vi "Switch - Making Connections on a Switch (NI-SWITCH).vi"() -> ()   [LabVIEW 2019]
doc: "I. Description:\n\nThis example demonstrates how to connect and disconnect channels. \n\n**Note that it is intended for use with matrix modules only, as multiplexer modules cannot connect more than one channel at a time. Using this VI with a multiplexer module will produce an error.**\n\nII. Instructions for Running:\n\nTo make this example work with your switch, complete the following:\n1 - Change Switch Resource Name and Topology Name as necessary.\n2 - Change Channel 1, 2, 3, and 4 to the names of the channels on your switch module. \n\nRefer to the NI Switches Help for the valid channel names and valid resource names for your switch module.\n\nIII. Block Diagram Steps:\n\n1 - Open session to switch module and set topology.\n2 - Connect specified channels.\n3 - Wait for relay(s) to activate and debounce.\n4 - Connect specified channels.\n5 - Wait for relay(s) to activate and debounce.\n6 - Disconnect all channels\n7 - Close session to switch module.\n8 - Display errors (if any).\n\nIV. I/O Connections Overview:\n\nRefer to the NI Switches Getting Started Guide and NI Switches Help for information about connecting signals to your switch module."
uses:
  <instrlib>/niSwitch/niSwitch.llb/niSwitch Topologies.ctl
  <instrlib>/niSwitch/niSwitch.llb/niSwitch Connect Channels (Multiple).vi
panel:
  in  "topology name":T1="Configured Topology" caption="Topology Name"
  in  "connection list2":string="[ab1->card1r1->c0]" caption="Channel 3"
  in  "connection list":string="[ab0->card1r0->c42]" caption="Channel 1"
  in  "resource name":refnum<k15>="2810_A1_SCSI1" caption="Resource Name"
  # "Note that this VI is intended for use with matrix modules only. \nFor further nstructions, select File >> VI Properties >> Documentation"
  # "Device Settings"
  # "First Connection"
  # "Second Connection"
  # "For a list of valid relay names, select \nHelp >> NI Switches Help >> Devices >> [Module Number]"
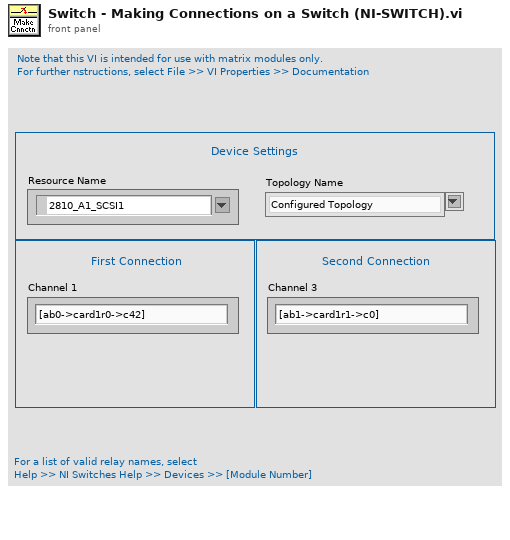
[diagram p1: front panel]
types:
  T1 = typedef "niSwitch Topologies.ctl" = string
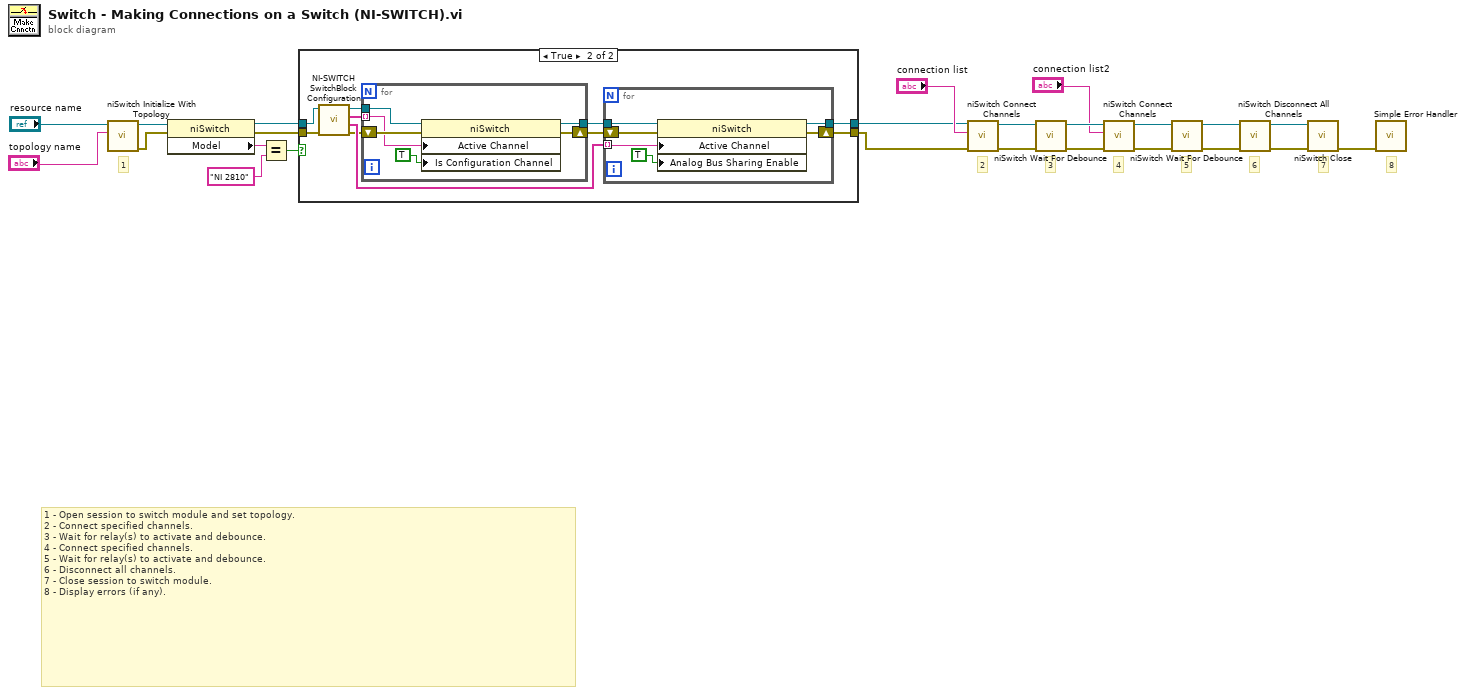
[diagram p0: block diagram]
diagram:
  # "8"
  # "4"
  # "5"
  # "7"
  # "3"
  # "6"
  # "2"
  # "1"
  # "1 - Open session to switch module and set topology.\n2 - Connect specified channels.\n3 - Wait for relay(s) to activate and debounce.\n4 - Connect specified channels.\n5 - Wait for relay(s) to activate and debounce.\n6 - Disconnect all channels. \n7 - Close session to switch module.\n8 - Display errors (if any)."
  n1 = call <instrlib>:"niSwitch Initialize With Topology.vi"("topology name"="topology name", "resource name"="resource name") -> ("error out"=w3:errorcluster, "instrument handle out"=w4:refnum<k15>)  [unwired: 3 in, 5 out]
  n2 = property class="niSwitch"(reference=w4, error in=w3) -> (reference out=w8:refnum<k15>, error out=w9:errorcluster, "Model"=w7:string)
  n3 = Equal?(x=w7, y="NI 2810") -> (x = y?=w5:bool)
  n4 = case shown="True" w5 {
    tunnel: [w26 w33] -> w2
    tunnel: [w25 w32] -> w1
    tunnel: w9 -> [w25 w30]
    tunnel: w8 -> [w26 w29]
    frame False {
    }
    frame True {
      n5 = call "NI-SWITCH SwitchBlock Configuration.vi"("error in (no error)"=w30, "Reference In"=w29) -> ("error out"=w27:errorcluster, "Analog Bus Array"=w28:string[], "Row Array"=w35:string[], "Reference out"=w31:refnum<k15>)  [unwired: 6 in]
      n6 = for {
        tunnel: w35 -> [w45] mode=indexing
        shift-right: [w47] -> w34
        shift-left: w27 -> [w46]
        tunnel: w31 -> [w44]
        tunnel: [w43] -> w36
        n7 = property class="niSwitch"(reference=w44, error in=w46, "Active Channel"=w45, "Is Configuration Channel"=TRUE ("Channel Configuration:Is Configuration Channel")) -> (reference out=w43:refnum<k15>, error out=w47:errorcluster)
      }
      n8 = for {
        shift-right: [w39] -> w32
        shift-left: w34 -> [w40]
        tunnel: w36 -> [w41]
        tunnel: [w38] -> w33
        tunnel: w28 -> [w37] mode=indexing
        n9 = property class="niSwitch"(reference=w41, error in=w40, "Active Channel"=w37, "Analog Bus Sharing Enable"=TRUE ("Channel Configuration:Is Configuration Channel")) -> (reference out=w38:refnum<k15>, error out=w39:errorcluster)
      }
    }
  }
  n10 = call-poly <instrlib>:"niSwitch Connect Channels.vi"("error in (no error)"=w1, "connection list"="connection list", "instrument handle"=w2) -> ("error out"=w23:errorcluster, "instrument handle out"=w22:refnum<k15>)  [unwired: 7 in]
  n11 = call <instrlib>:"niSwitch Wait For Debounce.vi"("error in (no error)"=w23, "instrument handle"=w22) -> ("error out"=w18:errorcluster, "instrument handle out"=w19:refnum<k15>)  [unwired: 1 in, 7 out]
  n12 = call-poly <instrlib>:"niSwitch Connect Channels.vi"("error in (no error)"=w18, "connection list"="connection list2", "instrument handle"=w19) -> ("error out"=w20:errorcluster, "instrument handle out"=w21:refnum<k15>)  [unwired: 7 in]
  n13 = call <instrlib>:"niSwitch Wait For Debounce.vi"("error in (no error)"=w20, "instrument handle"=w21) -> ("error out"=w12:errorcluster, "instrument handle out"=w13:refnum<k15>)  [unwired: 1 in, 7 out]
  n14 = call <instrlib>:"niSwitch Disconnect All Channels.vi"("error in (no error)"=w12, "instrument handle"=w13) -> ("error out"=w11:errorcluster, "instrument handle out"=w10:refnum<k15>)  [unwired: 8 in]
  n15 = call <instrlib>:"niSwitch Close.vi"("error in (no error)"=w11, "instrument handle"=w10) -> ("error out"=w24:errorcluster)  [unwired: 9 out]
  n16 = call <vilib>:"Simple Error Handler.vi"("error in (no error)"=w24) -> ()  [unwired: 1 in, 8 out]
